vi "제목없음 13.vi"   [LabVIEW 2020]
uses:
  <vilib>/Utility/sysdir.llb/System Directory Type.ctl
types:
  T1 = typedef "System Directory Type.ctl" = i32
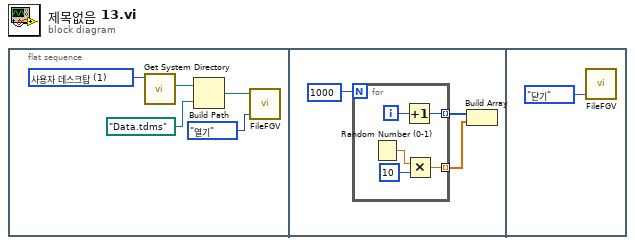
[diagram p0: block diagram]
diagram:
  n1 = flat-sequence {
    frame #0 {
      w2 = T1 1 items=["사용자 홈"=0, "사용자 데스크탑"=1, "사용자 문서"=2, "사용자 어플리케이션 데이터"=3, "사용자 환경"=4, "사용자 임시"=5, "퍼블릭 문서"=6, "퍼블릭 어플리케이션 데이터"=7, "퍼블릭 환경"=8, "퍼블릭 캐시"=13, "시스템 코어 라이브러리"=9, "시스템 설치된 라이브러리"=10, "어플리케이션 파일"=11, "부팅 볼륨 루트"=12] ("system directory type")
      n2 = call <vilib>:"Get System Directory.vi"("system directory type"=w2) -> ("system directory"=w4:path)  [unwired: 10 in]
      n3 = Build Path(base path=w4, name or relative path=path "Data.tdms" ("이름 또는 상대 경로")) -> (appended path=w5:path)
      n4 = call "FileFGV.vi"("File FGV 상태"=enum16{"열기", "쓰기", "닫기"}."열기", "파일 경로"=w5) -> ()  [unwired: 1 in]
    }
    frame #1 {
      n5 = for {
        N: 1000 -> [_]
        tunnel: [w12] -> w7 mode=indexing
        tunnel: [w9] -> w6 mode=indexing
        i -> [w13]
        n6 = Random Number (0-1)() -> (number: 0 to 1=w11:dbl)
        n7 = Increment(x=w13) -> (x+1=w12:i32)
        n8 = Multiply(x=w11, y=10) -> (x*y=w9:dbl)
      }
      n9 = Build Array(w7, w6) -> ()  [unwired: 1 out]
    }
    frame #2 {
      n10 = call "FileFGV.vi"("File FGV 상태"=enum16{"열기", "쓰기", "닫기"}."닫기") -> ()  [unwired: 2 in]
    }
  }
